vi "MICS, Telem Setup.vi"(6 "2.45 GHz Wake-Up Power (6)":i8(ring)=6 items=["-29"=-29, "-4"=-4, "-2"=-2, "0"=0, "2"=2, "4"=4, "6"=6, "8"=8, "10"=10, "12"=12, "14"=14, "16"=16, "18"=18, "20"=20, "22"=22, "24"=24, "26"=26, "27"=27], 8 "error in":errorcluster, 9 "Attenuation dB (0)":dbl, 10 "400 MHz MICS Power Setting (0x16)":u8=22 format="%02x", 11 "VISA resource":refnum<visa-resource-name>="COM9") -> (0 "error out":errorcluster, 3 "VISA resource dup":refnum<visa-resource-name>)   [LabVIEW 2020]
uses:
  Drivers/Telemetry/MICS Parameters Global.vi
  Drivers/Telemetry/MICS_Channel Global.vi
  Drivers/Telemetry/MICS_ID Global.vi
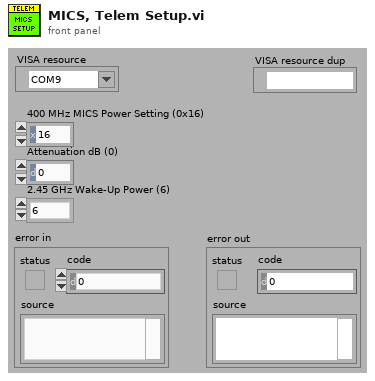
[diagram p1: front panel]
types:
  T1 = cluster{"ConfigFlags":u8, "ImplantID":u32, "CompanyID":u8, "Normal_Comm":cluster{"RF_Channel":u8, "UserData":u8, "TX_Mod":u8, "RX_Mod":u8, "RX_BlockSize":u8, "BlockPerPack":u8, "TX_BlockSize":u8}, "Emerg_Comm":cluster{"RF_Channel":u8, "UserData":u8, "TX_Mod":u8, "RX_Mod":u8, "TX_BlockSize":u8, "BlockPerPack":u8, "RX_BlockSize":u8}, "ImplantRev":u8, "245TX_PowerCal":i8, "245TX_Power":i8, "CCA_RSSI_Thresholds":cluster{"ch0":u16, "ch1":u16, "ch2":u16, "ch3":u16, "ch4":u16, "ch5":u16, "ch6":u16, "ch7":u16, "ch8":u16, "ch9":u16}}
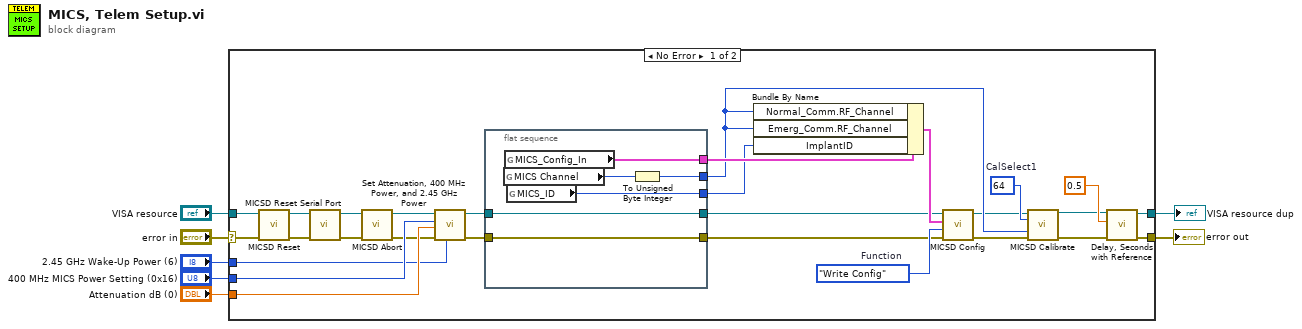
[diagram p0: block diagram]
diagram:
  n1 = case shown="No Error" "error in" {
    selector: "error in" -> [w30 w43]
    tunnel: "400 MHz MICS Power Setting (0x16)" -> [w23 _]
    tunnel: [w17 w43] -> w6
    tunnel: "VISA resource" -> [w31 w42]
    tunnel: "Attenuation dB (0)" -> [w24 _]
    tunnel: "2.45 GHz Wake-Up Power (6)" -> [w22 _]
    tunnel: [w18 w42] -> w1
    frame No Error {
      w29 = u8 64  # CalSelect1
      w28 = enum16{"Write Config", "Read Config"}."Write Config"  # Function
      n2 = call "MICSD Reset.vi"("error in (no error)"=w30, "VISA Resource Name"=w31) -> ("error out"=w35:errorcluster, "dup VISA Resource Name"=w34:refnum<visa-resource-name>)  [unwired: 8 in]
      n3 = call "MICSD Reset Serial Port.vi"("error in (no error)"=w35, "VISA Resource Name"=w34) -> ("error out"=w33:errorcluster, "dup VISA Resource Name"=w32:refnum<visa-resource-name>)  [unwired: 8 in]
      n4 = call "MICSD Abort.vi"("error in (no error)"=w33, "VISA Resource Name"=w32) -> ("error out"=w21:errorcluster, "dup VISA Resource Name"=w20:refnum<visa-resource-name>)  [unwired: 8 in]
      n5 = call "Set Attenuation, 400 MHz Power, and 2.45 GHz Power.vi"("2.45 GHz Wake-Up Power (6)"=w22, "error in"=w21, "Attenuation dB (0)"=w24, "400 MHz MICS Power Setting (0x16)"=w23, "VISA Resource Name"=w20) -> ("error out"=w12:errorcluster, "dup VISA Resource Name"=w13:refnum<visa-resource-name>)  [unwired: 5 in]
      n6 = flat-sequence {
        tunnel: [w41] -> w16
        tunnel: [w39] -> w14
        tunnel: [w38] -> w15
        tunnel: w13 -> [w37]
        tunnel: [w37] -> w9
        tunnel: w12 -> [w36]
        tunnel: [w36] -> w11
        frame #0 {
          n7 = global read "MICS_Channel Global.vi" "MICS Channel"() -> (w40:u16)
          n8 = global read "MICS Parameters Global.vi" "MICS_Config_In"() -> (w41:T1)
          n9 = global read "MICS_ID Global.vi" "MICS_ID"() -> (w38:u32)
          n10 = To Unsigned Byte Integer(number=w40) -> (unsigned 8bit integer=w39:u8)
        }
      }
      n11 = Bundle By Name(cluster=w16, "Normal_Comm.RF_Channel"=w14, "Emerg_Comm.RF_Channel"=w14, "ImplantID"=w15) -> (w27:T1)
      n12 = call "MICSD Config.vi"("error in (no error)"=w11, "Function"=w28, "MICS_Config_In"=w27, "VISA Resource Name"=w9) -> ("error out"=w10:errorcluster, "dup VISA Resource Name"=w8:refnum<visa-resource-name>)  [unwired: 5 in, 1 out]
      n13 = call "MICSD Calibrate.vi"("VISA Resource Name"=w8, "CalSelect1"=w29, "Channel"=w14, "error in (no error)"=w10) -> ("dup VISA Resource Name"=w19:refnum<visa-resource-name>, "error out"=w26:errorcluster)  [unwired: 10 in]
      n14 = call "Delay, Seconds with Reference.vi"("error in"=w26, "delay"=dbl[unit] 0.5, "VISA resource"=w19) -> ("error out"=w17:errorcluster, "VISA resource dup"=w18:refnum<visa-resource-name>)  [unwired: 3 in, 1 out]
    }
    frame Error {
    }
  }
  "error out" <- w6
  "VISA resource dup" <- w1
